vi "Get ROI.vi"(0 "Notifier Name":string, 11 "Error In":errorcluster) -> (4 "Notifier Name DUP":string, 8 "Camera ROI":T1, 15 "Error Out":errorcluster)   [LabVIEW 2020]
uses:
  Camera Controls/Generic Camera ROI.ctl
  Hardware Configuration/Hardware Configuration Controls/Company.ctl
  Hamamatsu/Orca Flash/Orca Flash Controls/Orca Flash Actions.ctl
  IDS/IDS Controls/IDS Actions.ctl
  Photometrics/Prime BSI/R Cubed SITK/Prime BSI R3 Controls/Prime R3 Actions.ctl
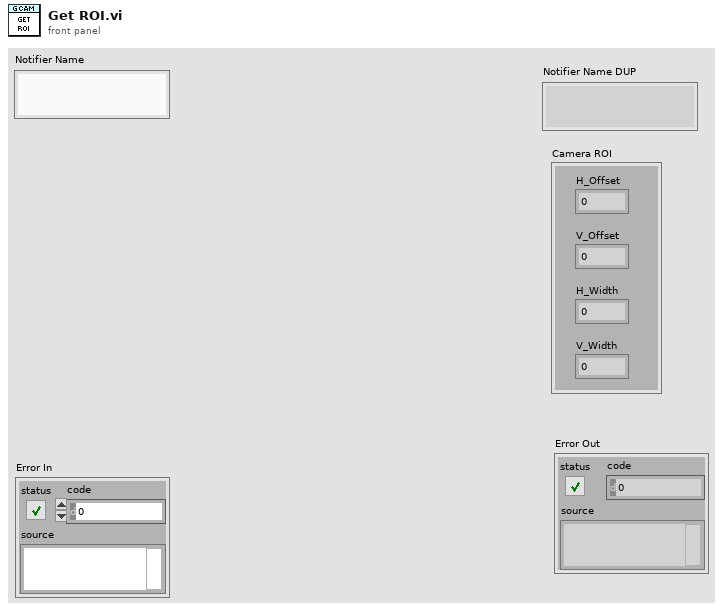
[diagram p1: front panel]
types:
  T1 = typedef "Generic Camera ROI.ctl" = cluster{"H_Offset":u16, "V_Offset":u16, "H_Width":u16, "V_Width":u16}
  T2 = typedef "Company.ctl" = enum16{"AA Opto Electronic", "ASI", "Coherent", "Creset Optics", "CVI", "DAQmx", "Hamamatsu", "IDS", "Mad City Labs", "Marzhauser", "Measurement Computing", "MPB Com", "Olympus", "Photometrics", "PI", "Prior", "Thorlabs"}
  T3 = typedef "Orca Flash Actions.ctl" = enum16{"Idle", "Preview", "Record", "Record Settings", "Set Param", "Get Param", "Set ROI", "Get ROI", "Trigger Source", "Trigger Type", "Progessive Mode", "Area Mode", "Status", "Quit"}
  T4 = typedef "IDS Actions.ctl" = enum16{"Error Check", "Initialize", "Preview", "Record", "Abort", "Record Settings", "Set Parameter", "Get Parameter", "Set ROI", "Get ROI", "Status", "Quit"}
  T5 = typedef "Prime R3 Actions.ctl" = enum16{"Error Check", "Initialize", "Preview", "Record", "Abort", "Record Settings", "Set Parameter", "Get Parameter", "Set ROI", "Get ROI", "Status", "Set Trigger", "Quit"}
  T6 = typedef "Orca Flash ROI.ctl" = cluster{"H Offset":i32, "V Offset":i32, "H Width":i32, "V Width":i32}
  T7 = typedef "IDS ROI.ctl" = cluster{"H Offset":i32, "V Offset":i32, "H Width":i32, "V Width":i32}
  T8 = typedef "Prime R3 ROI.ctl" = cluster{"X Start":u32, "X End":u32, "X Bin":u32, "Y Start":u32, "Y End":u32, "Y Bin":u32}
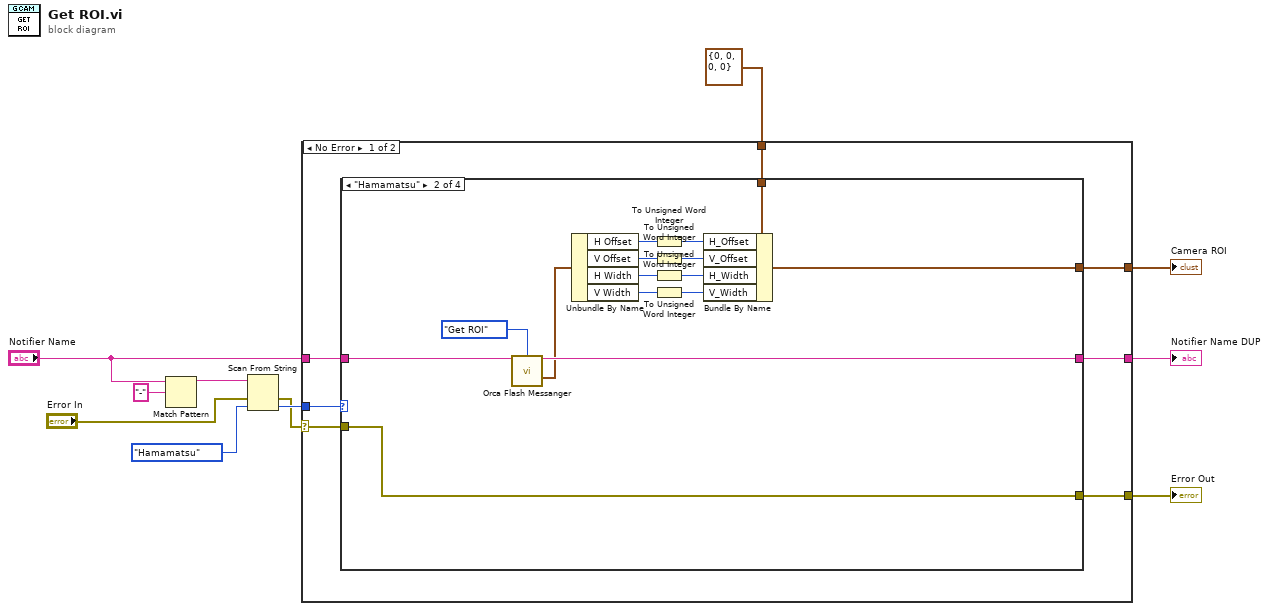
[diagram p0: block diagram]
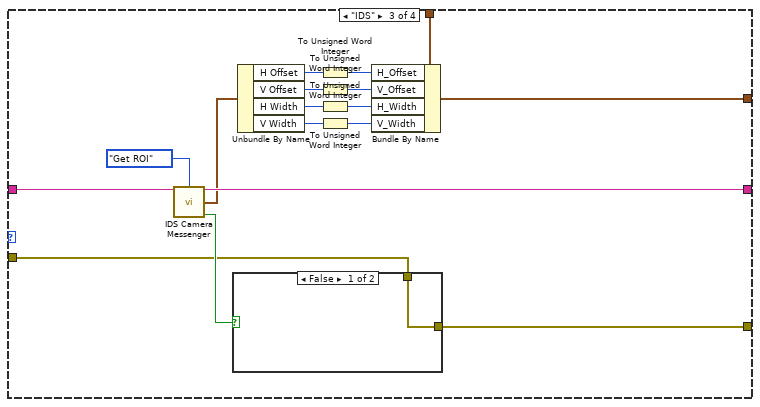
[diagram p3: hidden frame]
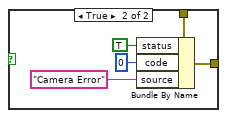
[diagram p4: hidden frame]
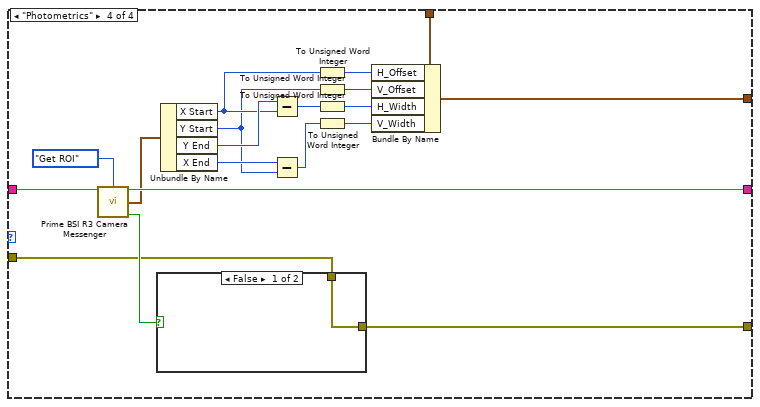
[diagram p5: hidden frame]
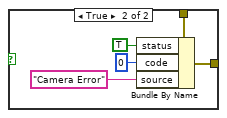
[diagram p6: hidden frame]
diagram:
  n1 = Match Pattern(string="Notifier Name", regular expression="-") -> (before substring=w9:string)  [unwired: 1 in, 3 out]
  n2 = Scan From String(input string=w9, error in="Error In", default 1=Company."Hamamatsu" ("Company")) -> (error out=w5:errorcluster, output 1=w8:T2)  [unwired: 2 in, 2 out]
  n3 = case shown="No Error" w5 {
    selector: w5 -> [w16 w86]
    tunnel: w8 -> [w18 _]
    tunnel: "Notifier Name" -> [w17 w87]
    tunnel: [w15 w87] -> w4
    tunnel: [w14 w86] -> w3
    tunnel: [w13 w85] -> w2
    tunnel: T1 {"H_Offset"=0, "V_Offset"=0, "H_Width"=0, "V_Width"=0} ("General Camera ROI") -> [w12 w85]
    frame No Error {
      n4 = case shown="\"Hamamatsu\"" w18 {
        tunnel: w17 -> [w21 w36 w53 w78]
        tunnel: w16 -> [w20 w34 w49 w75]
        tunnel: [w21 w35 w52 w77] -> w15
        tunnel: [w20 w34 w48 w74] -> w14
        tunnel: [w19 w24 w38 w71] -> w13
        tunnel: w12 -> [w19 w23 w37 w72]
        frame Default {
        }
        frame "Hamamatsu" {
          n5 = call "Orca Flash Messanger.vi"("Notifier Name"=w36, "Camera Actions"=Orca_Flash_Actions."Get ROI") -> ("Notifier Name Dup"=w35:string, "sCMOS ROI"=w25:T6)  [unwired: 9 in, 3 out]
          n6 = Unbundle By Name(w25) -> ("H Offset"=w33:i32, "V Offset"=w32:i32, "H Width"=w31:i32, "V Width"=w30:i32)
          n7 = To Unsigned Word Integer(number=w33) -> (unsigned 16bit integer=w29:u16)
          n8 = To Unsigned Word Integer(number=w32) -> (unsigned 16bit integer=w28:u16)
          n9 = To Unsigned Word Integer(number=w31) -> (unsigned 16bit integer=w27:u16)
          n10 = To Unsigned Word Integer(number=w30) -> (unsigned 16bit integer=w26:u16)
          n11 = Bundle By Name(cluster=w23, "H_Offset"=w29, "V_Offset"=w28, "H_Width"=w27, "V_Width"=w26) -> (w24:T1)
        }
        frame "IDS" {
          n12 = call "IDS Camera Messenger.vi"("Notifier Name"=w53, "IDS Actions"=IDS_Actions."Get ROI") -> ("Notifier Name (Dup)"=w52:string, "IDS ROI"=w39:T7, "Error?"=w50:bool)  [unwired: 8 in, 3 out]
          n13 = case shown="False" w50 {
            tunnel: w49 -> [w54 w59]
            tunnel: [w54 w58] -> w48
            frame False {
            }
            frame True {
              n14 = Bundle By Name(cluster=w59, "status"=TRUE, "code"=0, "source"="Camera Error") -> (w58:errorcluster)
            }
          }
          n15 = Unbundle By Name(w39) -> ("H Offset"=w47:i32, "V Offset"=w46:i32, "H Width"=w45:i32, "V Width"=w44:i32)
          n16 = To Unsigned Word Integer(number=w47) -> (unsigned 16bit integer=w43:u16)
          n17 = To Unsigned Word Integer(number=w46) -> (unsigned 16bit integer=w42:u16)
          n18 = To Unsigned Word Integer(number=w45) -> (unsigned 16bit integer=w41:u16)
          n19 = To Unsigned Word Integer(number=w44) -> (unsigned 16bit integer=w40:u16)
          n20 = Bundle By Name(cluster=w37, "H_Offset"=w43, "V_Offset"=w42, "H_Width"=w41, "V_Width"=w40) -> (w38:T1)
        }
        frame "Photometrics" {
          n21 = call "Prime BSI R3 Camera Messenger.vi"("Notifier Name"=w78, "Prime Actions"=Prime_R3_Actions."Get ROI") -> ("Notifier Name (Dup)"=w77:string, "Prime ROI"=w70:T8, "Error?"=w76:bool)  [unwired: 8 in, 3 out]
          n22 = case shown="False" w76 {
            tunnel: w75 -> [w79 w84]
            tunnel: [w79 w83] -> w74
            frame False {
            }
            frame True {
              n23 = Bundle By Name(cluster=w84, "status"=TRUE, "code"=0, "source"="Camera Error") -> (w83:errorcluster)
            }
          }
          n24 = Unbundle By Name(w70) -> ("X Start"=w66:u32, "Y Start"=w64:u32, "Y End"=w67:u32, "X End"=w65:u32)
          n25 = Subtract(x=w67, y=w66) -> (x-y=w63:u32)
          n26 = Subtract(x=w65, y=w64) -> (x-y=w62:u32)
          n27 = To Unsigned Word Integer(number=w66) -> (unsigned 16bit integer=w69:u16)
          n28 = To Unsigned Word Integer(number=w64) -> (unsigned 16bit integer=w68:u16)
          n29 = To Unsigned Word Integer(number=w63) -> (unsigned 16bit integer=w61:u16)
          n30 = To Unsigned Word Integer(number=w62) -> (unsigned 16bit integer=w60:u16)
          n31 = Bundle By Name(cluster=w72, "H_Offset"=w69, "V_Offset"=w68, "H_Width"=w61, "V_Width"=w60) -> (w71:T1)
        }
      }
    }
    frame Error {
    }
  }
  "Error Out" <- w3
  "Notifier Name DUP" <- w4
  "Camera ROI" <- w2
